vi "Direction to String.vi"(8 "error in (no error)":errorcluster, 11 "Halfwave Sinusoidal Fit in":refnum<class "Halfwave Sinusoidal Fit.lvclass">) -> (0 "error out":errorcluster, 2 "String":string, 3 "Halfwave Sinusoidal Fit out":refnum<class "Halfwave Sinusoidal Fit.lvclass">)   [LabVIEW 2013, in "Halfwave Sinusoidal Fit.lvclass"]
uses:
  Halfwave Sinusoidal Fit.lvclass
  Halfwave Sinusoidal Fit.lvclass/Halfwave Sinusoidal Fit.ctl
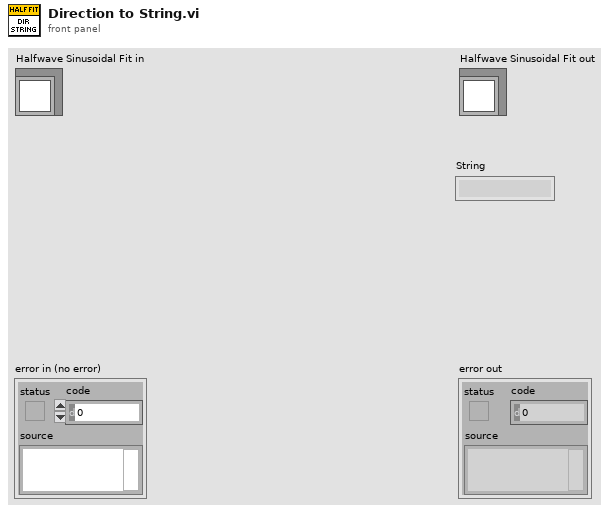
[diagram p1: front panel]
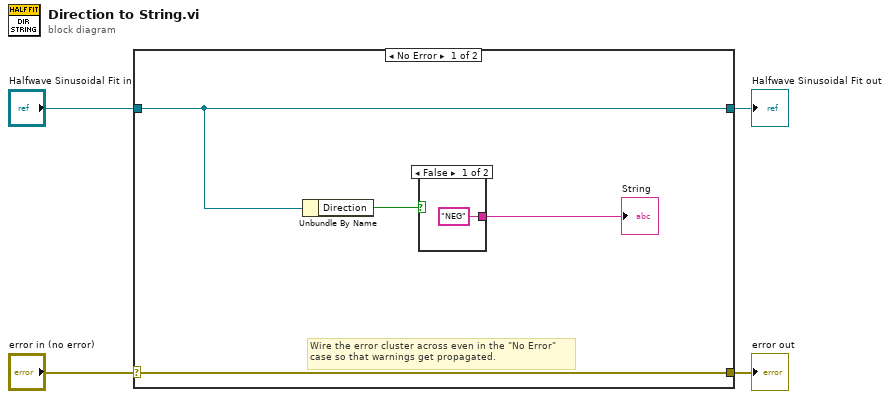
[diagram p0: block diagram]
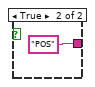
[diagram p2: hidden frame]
diagram:
  n1 = case shown="No Error" "error in (no error)" {
    selector: "error in (no error)" -> [w8 w12]
    tunnel: [w8 w12] -> w3
    tunnel: [w7 w11] -> w1
    tunnel: "Halfwave Sinusoidal Fit in" -> [w7 w11]
    frame No Error {
      # "Wire the error cluster across even in the \"No Error\"\ncase so that warnings get propagated."
      n2 = Unbundle By Name(w7) -> ("Direction"=w6:bool)
      n3 = case shown="False" w6 {
        tunnel: ["NEG" "POS"] -> w5
        frame False {
        }
        frame True {
        }
      }
      "String" <- w5
    }
    frame Error {
    }
  }
  "error out" <- w3
  "Halfwave Sinusoidal Fit out" <- w1
